vi "jMsg_TCPServer_Status - Rx Read.vi"(8 "error in (no error)":errorcluster, 11 "jModule":refnum<class "jModule.lvclass">) -> (0 "error out":errorcluster, 1 "Port":u16, 2 "Running?":bool, 3 "jModule":refnum<class "jModule.lvclass">, 7 "jMsg_TCPServer_Status":refnum<class "jMsg_TCPServer_Status.lvclass">)   [LabVIEW 2019, in "jMsg_TCPServer_Status.lvclass"]
doc: "This VI is used to read data from the jMsg\n\n\nJSMA Message Wizard 0.2.0.5\nRob Humfeld - Jet Engineering\nCopyright (c) 2020, Jet Engineering"
uses:
  jMsg_TCPServer_Status.lvclass
  <userlib>/Jet Engineering/JSMA/Libraries/jModule Class/jModule.lvclass
  <userlib>/Jet Engineering/JSMA/Libraries/jModule Class/jModule.lvclass/jModule.ctl
  jMsg_TCPServer_Status.lvclass/jMsg_TCPServer_Status.ctl
panel:
  in  "jMsg_TCPServer_Status":refnum<class "jMsg_TCPServer_Status.lvclass">
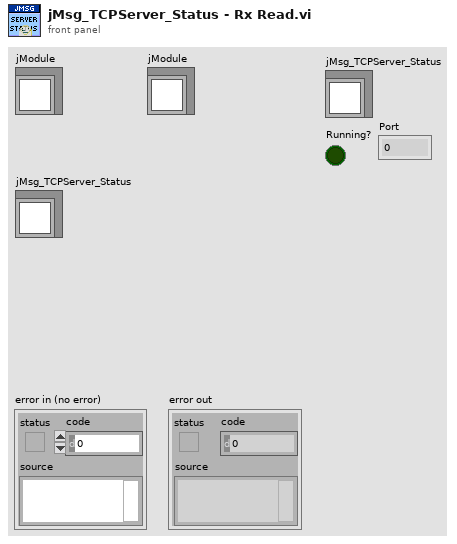
[diagram p1: front panel]
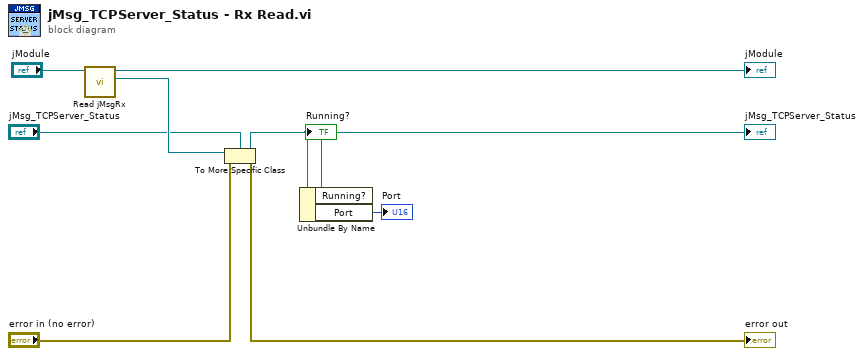
[diagram p0: block diagram]
diagram:
  n1 = call <userlib>:"Read jMsgRx.vi"("jModule in"="jModule") -> ("Received jMsg"=w6:refnum<class "jMsg.lvclass">, "jModule out"=→"jModule":refnum<class "jModule.lvclass">)  [unwired: 8 in, 1 out]
  n2 = To More Specific Class(target class="jMsg_TCPServer_Status", reference=w6, error in="error in (no error)") -> (specific class reference=w9:refnum<class "jMsg_TCPServer_Status.lvclass">, error out=→"error out":errorcluster)
  "jMsg_TCPServer_Status" <- w9
  n3 = Unbundle By Name(w9) -> ("Running?"=→"Running?":bool, "Port"=→"Port":u16)
